vi "Play Musicvi.vi"(8 "error in (no error)":errorcluster, 11 "Sound LUMP IN":u8[](array[numeric])=array[17283 elements]) -> (0 "error out":errorcluster)   [LabVIEW 2017]
panel:
  out "Output String":string
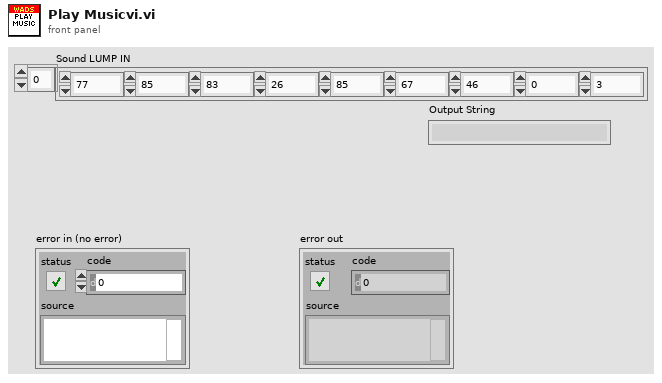
[diagram p1: front panel]
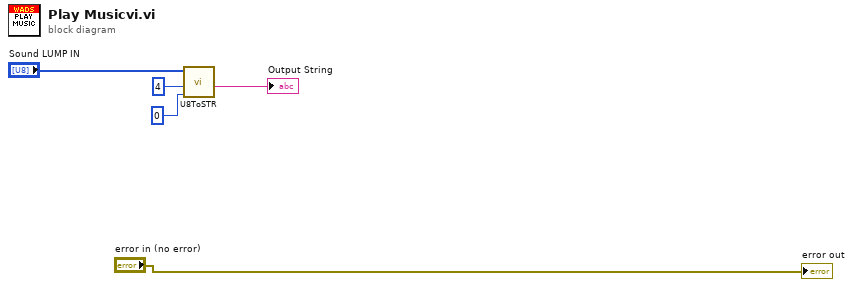
[diagram p0: block diagram]
diagram:
  n1 = call "U8ToSTR.vi"("Index"=u32 0, "Count"=4, "Input U8 Array"="Sound LUMP IN") -> ("Output String"=→"Output String":string)  [unwired: 2 in, 2 out]
  "error out" <- "error in (no error)"
